vi "Get Size of Data from TD - Enum U32 - Returns Correct Size.vi"() -> ()   [LabVIEW 2017, in "Composition.Tests.lvlib"]
uses:
  Composition.Tests.lvlib
  <vilib>/addons/_JKI Toolkits/Caraya/classes/Assert/Assert Equal Value_Variant.vi
  Composition/Composition.lvlib
  <vilib>/addons/_JKI Toolkits/Caraya/classes/Assert/Assert.lvclass
  <vilib>/addons/_JKI Toolkits/Caraya/classes/Test/Test.lvclass
panel:
  out "error out":errorcluster
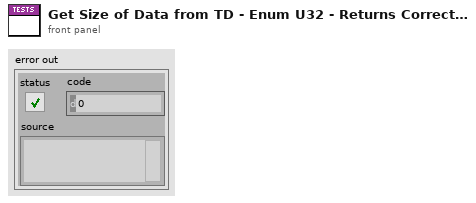
[diagram p1: front panel]
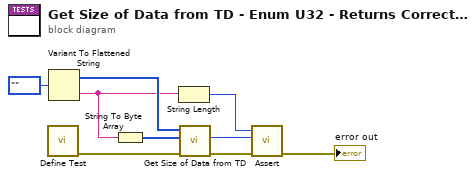
[diagram p0: block diagram]
diagram:
  n1 = call <vilib>:"Define Test.vi"() -> ("error out"=w1:errorcluster)  [unwired: 11 in]
  n2 = Variant To Flattened String(Variant=enum32{""}."") -> (data string=w5:string, 1:w9:i16[])
  n3 = String To Byte Array(string=w5) -> (unsigned byte array=w8:u8[])
  n4 = String Length(string=w5) -> (length=w2:i32)
  n5 = call "Get Size of Data from TD.vi"("error in (no error)"=w1, "Data String"=w8, "Type Descriptor"=w9) -> ("error out"=w7:errorcluster, "Size of Data"=w3:i32)  [unwired: 7 in]
  n6 = call-poly <vilib>:"Assert.vi"("error in (no error)"=w7, "Y"=w3, "X"=w2) -> ("error out"=→"error out":errorcluster)  [unwired: 8 in]
